vi "list - get closest string - V1.vi"(10 "number":i32, 11 "string Array":string[](array[string])) -> (0 "closest string":string, 1 "closest index":i32, 2 "closest value":i32)   [LabVIEW 2021]
uses:
  Q -- check range -- i -- real.vi
  Q - not nan -- real.vi
  <vilib>/regexp/Match Regular Expression.xnode
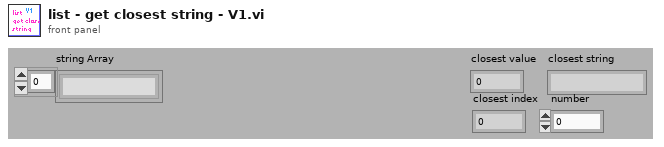
[diagram p1: front panel]
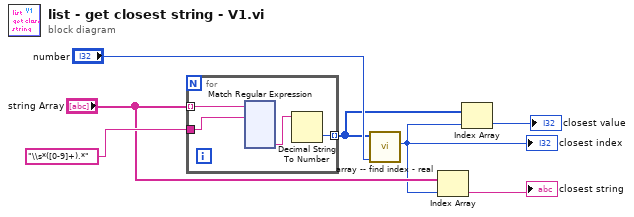
[diagram p0: block diagram]
diagram:
  n1 = for {
    tunnel: "\\s*([0-9]+).*" ("regular expression") -> [w11]
    tunnel: "string Array" -> [w10] mode=indexing
    tunnel: [w8] -> w3 mode=indexing
    n2 = xnode "Match Regular Expression"("input string"=w10, "regular expression"=w11) -> ("submatch 1"=w9:string)  [unwired: 4 in, 5 out]
    n3 = Decimal String To Number(string=w9) -> (number=w8:i32)  [unwired: 2 in, 1 out]
  }
  n4 = call "array -- find index - real.vi"("number"="number", "temperatures"=w3) -> ("closest element index"=w1:i32)  [unwired: 6 in, 3 out]
  "closest index" <- w1
  n5 = Index Array(array="string Array", index=w1) -> (element=→"closest string":string)
  n6 = Index Array(array=w3, index=w1) -> (element=→"closest value":i32)
